vi "Write Will Info.vi"(8 "error in (no error)":errorcluster, 10 "Will Info":T1={"Will Topic"="Will Topic", "Will message"="Last Will", "connMeta"={"qos"=enum."At most once", "duplicate"=FALSE, "retain"=TRUE}}, 11 "MQTT Client in":refnum<class "MQTT Client.lvclass">) -> (0 "error out":errorcluster, 3 "MQTT Client out":refnum<class "MQTT Client.lvclass">)   [LabVIEW 2020, in "MQTT Client.lvclass"]
uses:
  MQTT Client.lvclass
  mqttTypedef/WillDefinition.ctl
  mqttTypedef/ConnectionMeta.ctl
  mqttTypedef/QosLevel.ctl
  MQTT Client.lvclass/MQTT Client.ctl
  mqttCmd/BaseMqttMsg.lvclass
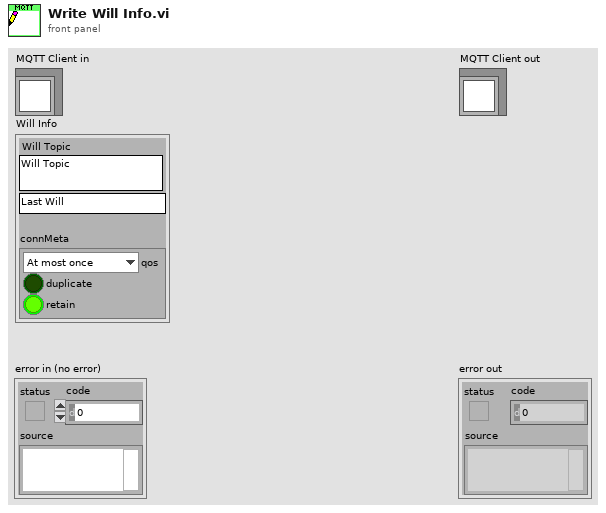
[diagram p1: front panel]
types:
  T1 = typedef "MQTT Client.lvclass/WillDefinition.ctl" = cluster{"Will Topic":string, "Will message":string, "connMeta":T2}
  T2 = typedef "MQTT Client.lvclass/ConnectionMeta.ctl" = cluster{"qos":T3, "duplicate":bool, "retain":bool}
  T3 = typedef "BaseMqttMsg.lvclass/QosLevel.ctl" = enum8{"At most once", "At least once", "Exactly once", "Reserved"}
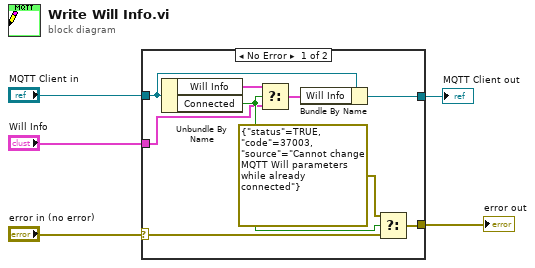
[diagram p0: block diagram]
diagram:
  n1 = case shown="No Error" "error in (no error)" {
    selector: "error in (no error)" -> [w12 w15]
    tunnel: [w11 w15] -> w1
    tunnel: [w14 w16] -> w4
    tunnel: "MQTT Client in" -> [w13 w16]
    tunnel: "Will Info" -> [w7 _]
    frame No Error {
      n2 = Unbundle By Name(w13) -> ("Will Info"=w9:T1, "Connected"=w8:bool)
      n3 = Select(t=w9, s=w8, f=w7) -> (s? t:f=w6:T1)
      n4 = Bundle By Name(cluster=w13, "Will Info"=w6) -> (w14:refnum<class "MQTT Client.lvclass">)
      n5 = Select(t=errorcluster {"status"=TRUE, "code"=37003, "source"="Cannot change MQTT Will parameters while already connected"}, s=w8, f=w12) -> (s? t:f=w11:errorcluster)
    }
    frame Error {
    }
  }
  "error out" <- w1
  "MQTT Client out" <- w4
